vi "Module Cleanup.vi"(8 "error in (no error)":errorcluster, 11 "Historian Logger in":refnum<class "Historian Logger.lvclass">) -> (0 "error out":errorcluster, 3 "Historian Logger out":refnum<class "Historian Logger.lvclass">)   [LabVIEW 2020, in "VolatusHistorian.lvlib" / "Historian Logger.lvclass"]
uses:
  Historian Logger.lvclass
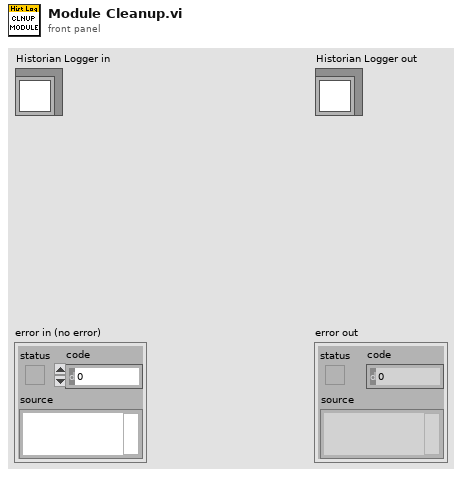
[diagram p1: front panel]
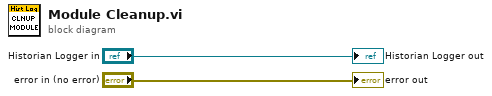
[diagram p0: block diagram]
diagram:
  "error out" <- "error in (no error)"
  "Historian Logger out" <- "Historian Logger in"
